vi "SVX Orbit and Timebase Plot (Unfiltered).vi"(0 "even-angle signals":cluster{"r0":dbl, "dr":dbl, "Y":dbl[]}[](array[cluster]) {"r0" format="%.2p"; "dr" format="%.2p"; "Y" format="%.2f"}, 2 "reset? (F)":bool, 5 "even-angle channel info":T1[](array[typedef]) {"channel info"."pregain" format="%.2f"; "channel info"."weighting filter" items=["Linear", "A-weighting", "B-weighting", "C-weighting", "ITU-R 468-4", "Dolby", "CCITT", "C-message", "Wb", "Wc", "Wd", "We", "Wf", "Wh", "Wj", "Wk", "Wm", "AES17 20 kHz lowpass", "AES17 40 kHz lowpass", "AES17 20 kHz highpass", "AES17 40 kHz highpass"]; "channel info"."dB reference" format="%^.1e"; "channel info"."engineering units" items=["custom..."=0, "V"=1, "A"=21, "C"=30, "pC"=31, "s"=32, "-"=29, "Pa"=2, "N"=20, "g"=3, "m/s^2"=4, "m/s"=5, "m"=6, "mm/s"=12, "mm"=13, "micron/s"=14, "micron"=15, "in/s^2"=7, "in/s"=8, "in"=9, "mil/s"=10, "mil"=11, "rad/s^2"=16, "rad/s"=17, "rad"=18, "deg/s^2"=26, "deg/s"=27, "deg"=28, "RPM"=22, "cycle/s^2"=23, "Hz"=24, "cycle"=25, "strain"=19]; "channel info"."sensor sensitivity" format="%#_5f"}, 7 "even-angle position info":T8, 9 "speed profile":T7 {"speed [RPM]" format="%.2f"; "time [s]" format="%.2f"}, 11 "error in (no error)":errorcluster, 12 "channel properties":T5[](array[typedef]) {"probe angle [deg]" max=360; "direction" items=["CCW", "CW"]}, 13 "segment settings":cluster{"start [rev]":dbl, "end [rev]":dbl}={"start [rev]"=0.0, "end [rev]"=inf}) -> (4 "orbit/timebase plot":T6(array[cluster]), 10 "end reached?":bool, 14 "actual segment settings":cluster{"start [rev]":dbl, "end [rev]":dbl}={"start [rev]"=0.0, "end [rev]"=inf}, 15 "error out":errorcluster)   [LabVIEW 2017, in "SoundVib_MCMDisplay.lvlib"]
doc: "Prepares unfiltered or filtered orbit plot data or timebase plot data for displaying on an Orbit Plot or Timebase Plot. Use this VI to prepare magnitude and phase data for entry into an orbit or timebase plot. Wire data to the <B>even-angle signals</B> input to determine the polymorphic instance to use or manually select the instance."
uses:
  <vilib>/addons/Sound and Vibration/Order Analysis/Data Presentation/SoundVib_MCMDisplay.lvlib
  <vilib>/addons/Sound and Vibration/Order Analysis/Misc/OAT Position Info.ctl
  <vilib>/addons/Sound and Vibration/Order Analysis/Tach Process/SubVIs/speed profile.ctl
  <vilib>/addons/Sound and Vibration/Order Analysis/Data Presentation/SubVIs/OAT MCM Channel Property.ctl
  <vilib>/addons/_NISVFA/_Shared subVIs/Controls/svc_Resampled Channel Info.ctl
  <vilib>/addons/_NISVFA/_Shared subVIs/Controls/svc_Channel Info.ctl
  <vilib>/addons/_NISVFA/_Shared subVIs/Controls/svc_Engineering Units Text Ring.ctl
  <vilib>/addons/_NISVFA/_Shared subVIs/Controls/svc_Weighting Filter Text Ring.ctl
  <vilib>/addons/Sound and Vibration/Order Analysis/Resample Order Tracking/SoundVib_Resampling.lvlib
  <vilib>/addons/Sound and Vibration/Order Analysis/Tach Process/SoundVib_TachProcess.lvlib
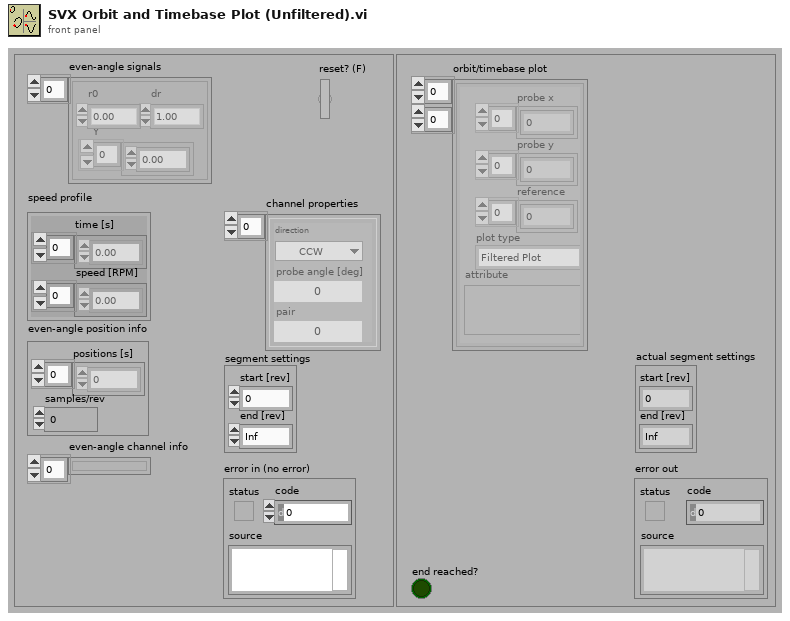
[diagram p1: front panel]
types:
  T1 = typedef "svc_Resampled Channel Info.ctl" = cluster{"channel name":string, "description":string, " channel info":T2}
  T2 = typedef "svc_Channel Info.ctl" = cluster{"sensor sensitivity":dbl, "engineering units":T3, "dB reference":dbl, "custom label":string, "weighting filter":T4, "pregain":dbl}
  T3 = typedef "svc_Engineering Units Text Ring.ctl" = u16
  T4 = typedef "svc_Weighting Filter Text Ring.ctl" = u16
  T5 = typedef "OAT MCM Channel Property.ctl" = cluster{"direction":u16, "probe angle [deg]":u16, "pair":u16}
  T6 = cluster{"probe x":dbl[], "probe y":dbl[], "reference":dbl[], "plot type":enum16{"Filtered Plot", "Unfiltered Plot"}, "attribute":variant}[][]
  T7 = typedef "SoundVib_TachProcess.lvlib/speed profile.ctl" = cluster{"time [s]":dbl[], "speed [RPM]":dbl[]}
  T8 = typedef "OAT Position Info.ctl" = cluster{"positions [s]":dbl[], "samples/rev":dbl}
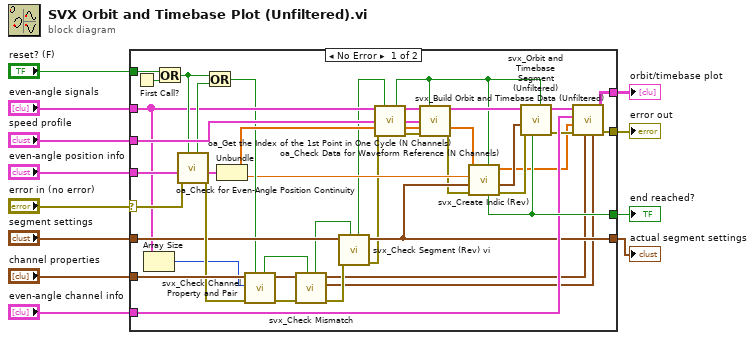
[diagram p0: block diagram]
diagram:
  n1 = case shown="No Error" "error in (no error)" {
    selector: "error in (no error)" -> [w50 w56]
    tunnel: [w45 w56] -> w11
    tunnel: "even-angle signals" -> [w39 _]
    tunnel: "speed profile" -> [w55 _]
    tunnel: "even-angle position info" -> [w49 _]
    tunnel: "reset? (F)" -> [w52 _]
    tunnel: "channel properties" -> [w46 _]
    tunnel: [w44 _] -> w5
    tunnel: "segment settings" -> [w42 _]
    tunnel: [w41 _] -> w3
    tunnel: "even-angle channel info" -> [w40 _]
    tunnel: [w35 _] -> w1
    frame No Error {
      n2 = First Call?() -> (First Call?: T/F=w53:bool)
      n3 = Array Size(array=w39) -> (size(s)=w37:i32)
      n4 = Or(x=w52, y=w53) -> (x .or. y?=w47:bool)
      n5 = call <vilib>:"oa_Check for Even-Angle Position Continuity.vi"("reset in"=w47, "error in (no error)"=w50, "even-angle position info"=w49) -> ("error out"=w43:errorcluster, "even-angle position info dup"=w48:T8, "position not continuous"=w51:bool)  [unwired: 6 in]
      n6 = Or(x=w47, y=w51) -> (x .or. y?=w38:bool)
      n7 = Unbundle(w48) -> ("positions [s]"=w54:dbl[], "samples/rev"=w36:dbl)
      n8 = call <vilib>:"svx_Check Channel Property and Pair.vi"("reset in"=w38, "error in (no error)"=w43, "channel number"=w37, "channel property"=w46) -> ("error out"=w20:errorcluster, "channel property out"=w18:T5[], "reset out"=w14:bool)  [unwired: 5 in]
      n9 = call <vilib>:"svx_Check Mismatch.vi"("reset in"=w14, "error in (no error)"=w20, "channel property in"=w18) -> ("error out"=w19:errorcluster, "pair index"=w16:cluster{"index 1":i32, "index 2":i32}[], "channel property out"=w17:T5[], "reset out"=w13:bool)  [unwired: 5 in]
      n10 = call <vilib>:"svx_Check Segment (Rev) vi.vi"("reset in"=w13, "error in (no error)"=w19, "segment settings"=w42) -> ("error out"=w27:errorcluster, "actual segment settings"=w35:cluster{"start [rev]":dbl, "end [rev]":dbl}, "reset out"=w15:bool)  [unwired: 6 in]
      n11 = call <vilib>:"oa_Check Data for Waveform Reference (N Channels).vi"("resampled signal"=w39, "reset? (True)"=w15, "speed profile"=w55, "interpolated pulse positions"=w54, "error in (no error)"=w27) -> ("reset"=w21:bool, "resampled data out"=w33:cluster{"r0":dbl, "dr":dbl, "Y":dbl[]}[], "speed profile out"=w31:T7, "interpolated pulse positions out"=w32:dbl[], "error out"=w34:errorcluster)  [unwired: 3 in, 3 out]
      n12 = call <vilib>:"oa_Get the Index of the 1st Point in One Cycle (N Channels).vi"("resampled signal"=w33, "reset? (True)"=w21, "speed profile"=w31, "interpolated pulse positions"=w32, "error in (no error)"=w34) -> ("resampled signal out"=w30:cluster{"r0":dbl, "dr":dbl, "Y":dbl[]}[], "interpolated pulse positions out"=w25:dbl[], "error out"=w26:errorcluster)  [unwired: 8 in]
      n13 = call <vilib>:"svx_Create Indic (Rev).vi"("reset?(F)"=w21, "error in (no error)"=w26, "segment settings"=w35, "actual samples/rev"=w36, "interpolated pulse positions in"=w25) -> ("error out"=w24:errorcluster, "indice"=w23:cluster{"start":i32, "length":i32}, "interpolated pulse positions out"=w22:dbl[], "end reached"=w41:bool)  [unwired: 2 in, 1 out]
      n14 = call <vilib>:"svx_Orbit and Timebase Segment (Unfiltered).vi"("reset? (F)"=w21, "end reach?"=w41, "error in (no error)"=w24, "indice"=w23, "resampled signal in"=w30) -> ("error out"=w28:errorcluster, "resampled signal out"=w29:cluster{dbl[], dbl}[])  [unwired: 5 in]
      n15 = call <vilib>:"svx_Build Orbit and Timebase Data (Unfiltered).vi"("pair index"=w16, "channel properties"=w17, "error in (no error)"=w28, "interpolated pulse positions[s]"=w22, "even-angle channel info"=w40, "resampled signal out"=w29) -> ("error out"=w45:errorcluster, "orbit/timebase plot"=w44:T6)  [unwired: 4 in]
    }
    frame Error {
    }
  }
  "error out" <- w11
  "orbit/timebase plot" <- w5
  "end reached?" <- w3
  "actual segment settings" <- w1
